vi "Timer FGV.vi"(8 "error in (no error)":errorcluster, 11 "Enum":T1) -> (0 "error out":errorcluster, 3 "Elapsed Time":dbl)   [LabVIEW 2017, in "admittanceControllerLibrary.lvlib"]
doc: "This is the timer required to generate intermediate points for the minimum jerk trajectory"
uses:
  admittanceControllerLibrary.lvlib
  Controls/timer control.ctl
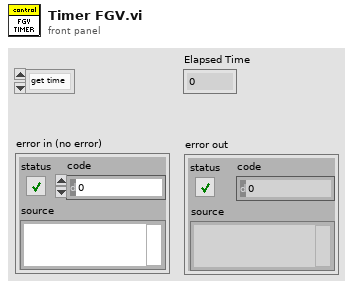
[diagram p1: front panel]
types:
  T1 = typedef "admittanceControllerLibrary.lvlib/timer control.ctl" = enum16{"get time", "set time"}
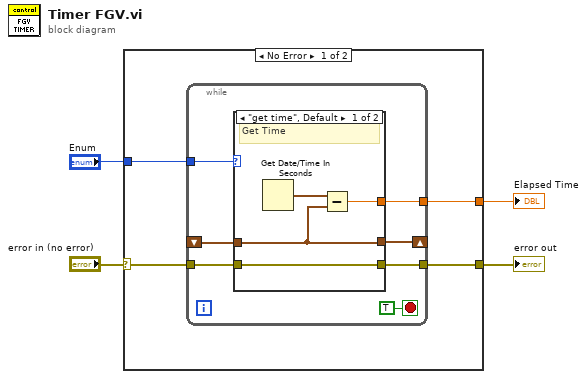
[diagram p0: block diagram]
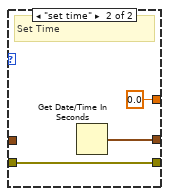
[diagram p2: hidden frame]
diagram:
  n1 = case shown="No Error" "error in (no error)" {
    selector: "error in (no error)" -> [w6 w23]
    tunnel: [w8 _] -> w4
    tunnel: "Enum" -> [w7 _]
    tunnel: [w5 w23] -> w1
    frame No Error {
      n2 = while {
        tunnel: w7 -> [w14]
        shift-right: [w13] -> _
        shift-left: _ -> [w12]
        tunnel: [w11] -> w8
        tunnel: w6 -> [w10]
        tunnel: [w9] -> w5
        stop <- TRUE stop-if-true
        n3 = case shown="\"get time\", Default" w14 {
          tunnel: [w18 w22] -> w13
          tunnel: w12 -> [w18 _]
          tunnel: [w17 0.0] -> w11
          tunnel: w10 -> [w16 w20]
          tunnel: [w16 w20] -> w9
          frame "get time", Default {
            # "Get Time"
            n4 = Get Date/Time In Seconds() -> (seconds since 1Jan1904=w19:timestamp)
            n5 = Subtract(x=w19, y=w18) -> (x-y=w17:dbl)
          }
          frame "set time" {
            # "Set Time"
            n6 = Get Date/Time In Seconds() -> (seconds since 1Jan1904=w22:timestamp)
          }
        }
      }
    }
    frame Error {
    }
  }
  "Elapsed Time" <- w4
  "error out" <- w1
